vi "Marker Input.vi"(8 "error in (no error)":errorcluster, 11 "Data In":T1 {"Toggle Channels"."Initial State" items=["High"=101, "Low"=102]; "Sample Rate" format="%.2p"}) -> (0 "error out":errorcluster, 3 "Data Out":T1 {"Toggle Channels"."Initial State" items=["High"=101, "Low"=102]; "Sample Rate" format="%.2p"})   [LabVIEW 2021]
uses:
  Controls/Data.ctl
  Controls/Script Trigger Routing.ctl
  Controls/Toggle Channel.ctl
  <instrlib>/niFgen/niFgen.llb/niFgen_ctl Exported Signal Name Values (Ring).ctl
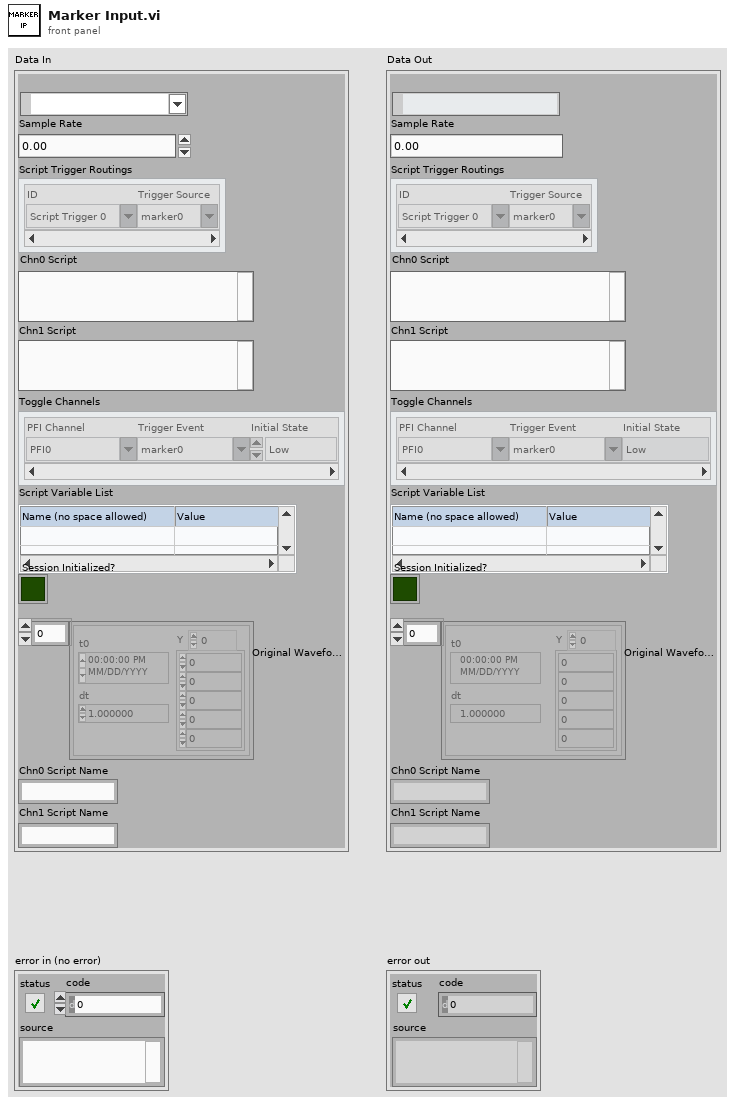
[diagram p1: front panel]
types:
  T1 = typedef "Data.ctl" = cluster{"FGEN Resource Name":refnum<k15>, "Sample Rate":dbl, "Script Trigger Routings":T2[], "Chn0 Script":string, "Chn1 Script":string, "Toggle Channels":T3[], "Script Variable List":string[][], "Session Initialized?":bool, "Original Waveforms":waveform(dbl)[], "Chn0 Script Name":string, "Chn1 Script Name":string}
  T2 = typedef "Script Trigger Routing.ctl" = cluster{"ID":string, "Trigger Source":string}
  T3 = typedef "Toggle Channel.ctl" = cluster{"PFI Channel":string, "Trigger Event":string, "Initial State":u16}
  T4 = typedef "niFgen_ctl Exported Signal Name Values (Ring).ctl" = u16
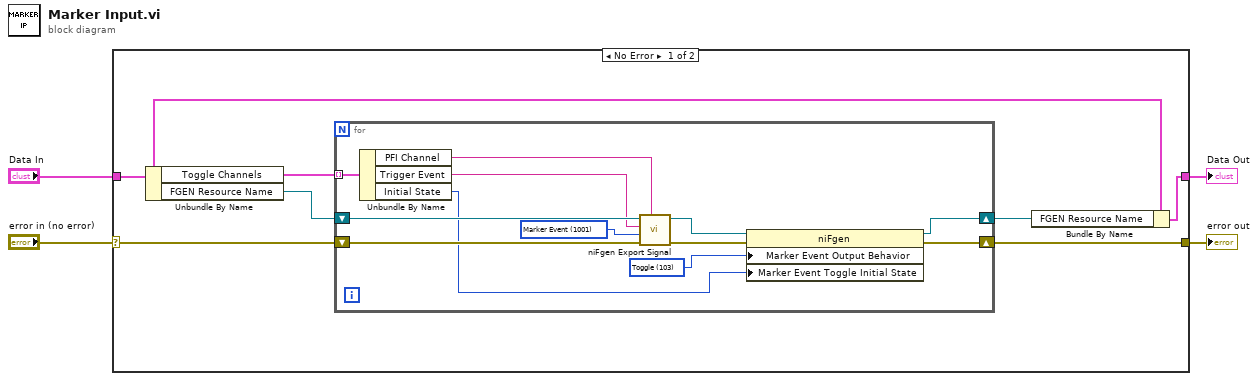
[diagram p0: block diagram]
diagram:
  n1 = case shown="No Error" "error in (no error)" {
    selector: "error in (no error)" -> [w8 w25]
    tunnel: "Data In" -> [w11 w24]
    tunnel: [w10 w24] -> w3
    tunnel: [w6 w25] -> w1
    frame No Error {
      n2 = Unbundle By Name(w11) -> ("Toggle Channels"=w5:T3[], "FGEN Resource Name"=w9:refnum<k15>)
      n3 = for {
        shift-right: [w17] -> w7
        shift-left: w9 -> [w23]
        shift-right: [w16] -> w6
        shift-left: w8 -> [w19]
        tunnel: w5 -> [w15] mode=indexing
        w18 = 103 items=["Pulse"=101, "Toggle"=103] ("Events:Marker:Output Behavior")
        w22 = T4 1001 items=["Sample Clock"=101, "Sample Clock Timebase"=1006, "Reference Clock"=102, "Onboard Reference Clock"=1019, "Start Trigger"=1004, "Script Trigger"=103, "Marker Event"=1001, "Data Marker Event"=108, "Ready For Start Event"=105, "Started Event"=106, "Done Event"=107, "Synchronization Pulse"=1007, "Sync Out"=1002] ("Signal")
        n4 = Unbundle By Name(w15) -> ("PFI Channel"=w14:string, "Trigger Event"=w13:string, "Initial State"=w12:u16)
        n5 = call <instrlib>:"niFgen Export Signal.vi"("Output Terminal (do not export)"=w14, "error in (no error)"=w19, "Signal"=w22, "Signal Identifier (None)"=w13, "Instrument Handle"=w23) -> ("error out"=w20:errorcluster, "Instrument Handle Out"=w21:refnum<k15>)  [unwired: 5 in]
        n6 = property class="niFgen"(reference=w21, error in=w20, "Marker Event Output Behavior"=w18, "Marker Event Toggle Initial State"=w12) -> (reference out=w17:refnum<k15>, error out=w16:errorcluster)
      }
      n7 = Bundle By Name(cluster=w11, "FGEN Resource Name"=w7) -> (w10:T1)
    }
    frame Error {
    }
  }
  "Data Out" <- w3
  "error out" <- w1
